vi "Build Context Menu.vi"(0 "FSM.Graph in":T2, 5 "Display State In in":T3, 7 "MenuRef":refnum<k9>, 9 "Coords":T1) -> (4 "FSM.Graph out":T2, 6 "Display State In out":T3)   [LabVIEW 2015, in "FSM Editor.xctl"]
uses:
  FSM Editor.xctl
  State.vi
  Classes/FSM.Port/FSM.Port.lvclass
  <vilib>/Utility/miscctls.llb/LVPoint32TypeDef.ctl
  Drag Mode.ctl
  Events.ctl
  NodeAdded.ctl
  NodeSelected.ctl
  EdgeEventData.ctl
  Data.vi
  Classes/FSM.Graph/FSM.Graph.lvclass
  Classes/FSM.Graph/FSM.Graph.lvclass/FSM.Graph.ctl
  Classes/FSM.Node/Shape.ctl
  Classes/FSM.Node/FSM.Node.lvclass/FSM.Node.ctl
  Classes/FSM.Node/Read Name.vi
  Classes/FSM.Node/Read Shape.vi
  Classes/FSM.Graph/Read selectedNodes.vi
  Classes/FSM.Graph/Read selectedEdge.vi
  Classes/FSM.Node/FSM.Node.lvclass
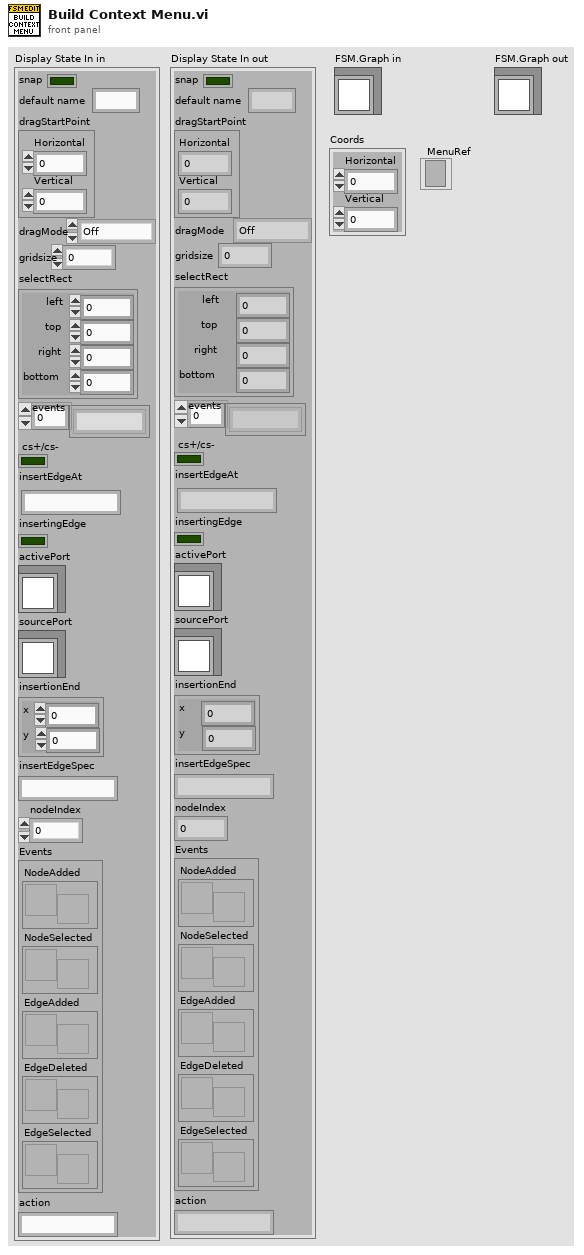
[diagram p1: front panel]
types:
  T1 = typedef "LVPoint32TypeDef.ctl" = cluster{"Horizontal":i32, "Vertical":i32}
  T2 = typedef "FSM Editor.xctl/Data.vi" = refnum<class "FSM.Graph.lvclass">
  T3 = typedef "FSM Editor.xctl/State.vi" = cluster{"snap":bool, "default name":string, "dragStartPoint":T1, "dragMode":T4, "gridsize":dbl, "selectRect":cluster{"left":i16, "top":i16, "right":i16, "bottom":i16}, "events":string[], "cs+/cs-":bool, "insertEdgeAt":string, "insertingEdge":bool, "activePort":refnum<class "FSM.Port.lvclass">, "sourcePort":refnum<class "FSM.Port.lvclass">, "insertionEnd":cluster{"x":i16, "y":i16}, "insertEdgeSpec":string, "nodeIndex":i32, "Events":T5, "action":string}
  T4 = typedef "Drag Mode.ctl" = enum16{"Off", "NodePending", "Nodes", "Pan", "Select", "EdgeInsertion", "EdgePoint", "EdgeLabel"}
  T5 = typedef "FSM Editor.xctl/Events.ctl" = cluster{"NodeAdded":refnum<user-event>, "NodeSelected":refnum<user-event>, "EdgeAdded":refnum<user-event>, "EdgeDeleted":refnum<user-event>, "EdgeSelected":refnum<user-event>}
  T6 = typedef "FSM.Node.lvclass/Shape.ctl" = enum16{"Default", "Start", "Action", "End"}
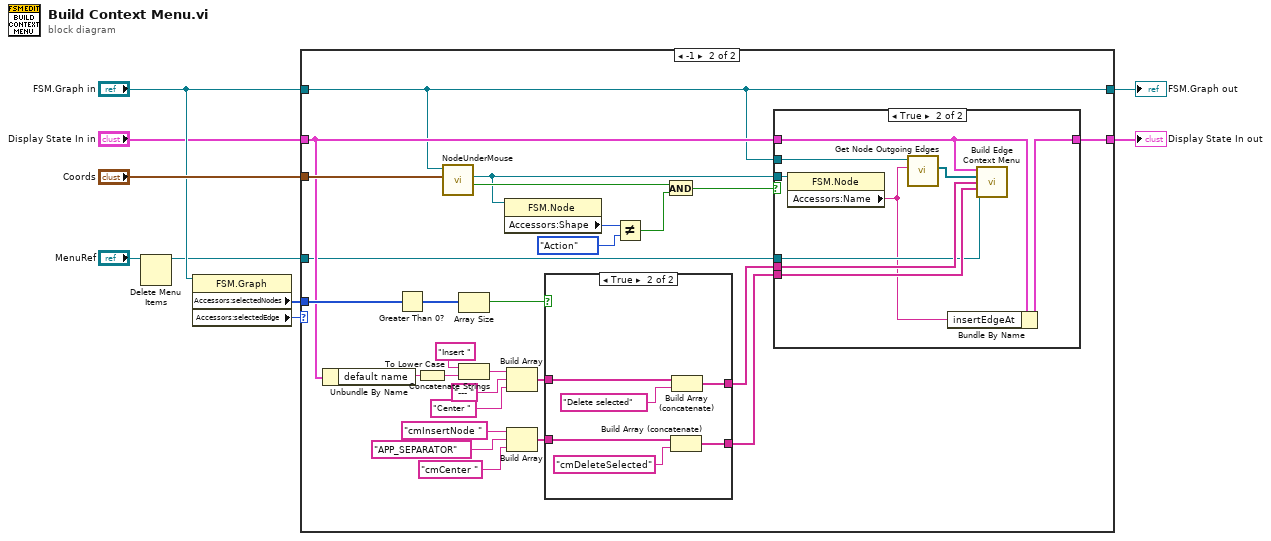
[diagram p0: block diagram]
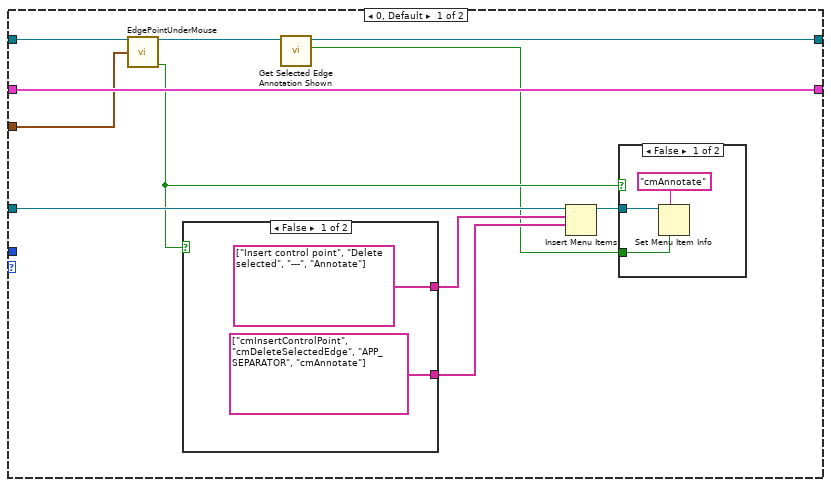
[diagram p2: hidden frame]
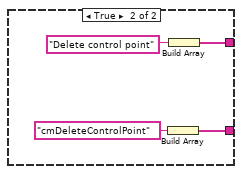
[diagram p4: hidden frame]
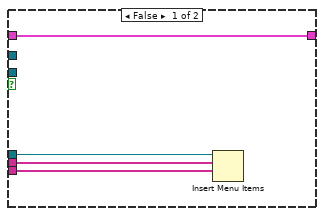
[diagram p5: hidden frame]
diagram:
  n1 = Delete Menu Items(9:"MenuRef") -> (3:w3:refnum<k9>)  [unwired: 3 in, 1 out]
  n2 = property class="FSM.Graph"(reference="FSM.Graph in") -> ("Accessors:selectedNodes"=w8:i32[], "Accessors:selectedEdge"=w2:i32)  [unwired: 1 in, 2 out]
  n3 = case shown="-1" w2 {
    tunnel: w8 -> [_ w54]
    tunnel: "Coords" -> [w16 w46]
    tunnel: "FSM.Graph in" -> [w13 w39]
    tunnel: [w20 w45] -> w5
    tunnel: "Display State In in" -> [w20 w44]
    tunnel: w3 -> [w19 w41]
    tunnel: [w11 w39] -> w1
    frame 0, Default {
      n4 = call "EdgePointUnderMouse.vi"("FSM.Graph In"=w13, "Coords"=w16) -> ("FSM.Graph Out"=w12:T2, "edge point?"=w14:bool)  [unwired: 12 in]
      n5 = case shown="False" w14 {
        tunnel: [string[] ["Insert control point", "Delete selected", "---", "Annotate"] w27] -> w18
        tunnel: [string[] ["cmInsertControlPoint", "cmDeleteSelectedEdge", "APP_SEPARATOR", "cmAnnotate"] w26] -> w17
        frame False {
        }
        frame True {
          n6 = Build Array("cmDeleteControlPoint" ("string")) -> (w26:string[])
          n7 = Build Array("Delete control point" ("string")) -> (w27:string[])
        }
      }
      n8 = call "Get Selected Edge Annotation Shown.vi"("FSM in"=w12) -> ("shown"=w10:bool, "FSM out"=w11:T2)  [unwired: 8 in, 1 out]
      n9 = Insert Menu Items(7:w17, 8:w18, 9:w19) -> (3:w15:refnum<k9>)  [unwired: 3 in, 2 out]
      n10 = case shown="False" w14 {
        tunnel: w15 -> [w23 _]
        tunnel: w10 -> [w21 _]
        frame False {
          n11 = Set Menu Item Info(6:w21, 7:"cmAnnotate" ("item tag"), 11:w23) -> ()  [unwired: 4 in, 2 out]
        }
        frame True {
        }
      }
    }
    frame -1 {
      n12 = Unbundle By Name(w44) -> ("default name"=w56:string)
      n13 = To Lower Case(string=w56) -> (all lower case string=w47:string)
      n14 = call "NodeUnderMouse.vi"("Coords"=w46, "FSM in"=w39) -> ("contains mouse"=w40:bool, "Node"=w38:refnum<class "FSM.Node.lvclass">)  [unwired: 6 in, 2 out]
      n15 = Array Size(array=w54) -> (size(s)=w52:i32)
      n16 = Greater Than 0?(x=w52) -> (x > 0?=w53:bool)
      n17 = Concatenate Strings("Insert " ("string"), w47) -> (w51:string)
      n18 = property class="FSM.Node"(reference=w38) -> ("Accessors:Shape"=w37:T6)  [unwired: 1 in, 2 out]
      n19 = Build Array(w51, "--- " ("string"), "Center " ("string")) -> (w49:string[])
      n20 = Build Array("cmInsertNode " ("string"), "APP_SEPARATOR", "cmCenter " ("string")) -> (w48:string[])
      n21 = case shown="True" w53 {
        tunnel: w49 -> [w71 w77]
        tunnel: w48 -> [w70 w75]
        tunnel: [w71 w73] -> w43
        tunnel: [w70 w72] -> w42
        frame False {
        }
        frame True {
          n22 = Build Array (concatenate)(w75, "cmDeleteSelected" ("string")) -> (w72:string[])
          n23 = Build Array (concatenate)(w77, "Delete selected" ("string")) -> (w73:string[])
        }
      }
      n24 = Not Equal?(x=w37, y=Shape."Action") -> (x != y?=w35:bool)
      n25 = And(x=w40, y=w35) -> (x .and. y?=w36:bool)
      n26 = case shown="True" w36 {
        tunnel: [w60 w65] -> w45
        tunnel: w44 -> [w60 w66]
        tunnel: w38 -> [_ w64]
        tunnel: w43 -> [w58 w69]
        tunnel: w42 -> [w57 w68]
        tunnel: w41 -> [w59 w67]
        tunnel: w39 -> [_ w63]
        frame False {
          n27 = Insert Menu Items(7:w57, 8:w58, 9:w59) -> ()  [unwired: 3 in, 3 out]
        }
        frame True {
          n28 = property class="FSM.Node"(reference=w64) -> ("Accessors:Name"=w62:string)  [unwired: 1 in, 2 out]
          n29 = call "Get Node Outgoing Edges.vi"("Name"=w62, "FSM in"=w63) -> ("Edges"=w61:refnum<class "FSM.Edge.lvclass">[])  [unwired: 7 in, 2 out]
          n30 = Bundle By Name(cluster=w66, "insertEdgeAt"=w62) -> (w65:T3)
          n31 = call "Build Edge Context Menu.vi"("Display State In"=w66, "Edges"=w61, "Names"=w69, "Tags"=w68, "menu ref"=w67) -> ()  [unwired: 11 in]
        }
      }
    }
  }
  "Display State In out" <- w5
  "FSM.Graph out" <- w1
